vi "GETPINSTATUS.vi"(8 "error in (no error)":errorcluster, 9 "pin":dbl, 10 "Port":dbl, 11 "simulado in":refnum<class "simulado.lvclass">) -> (0 "error out":errorcluster, 3 "simulado out":refnum<class "simulado.lvclass">)   [LabVIEW 2019, in "simulado.lvclass"]
uses:
  simulado.lvclass
  simulado.lvclass/simulado.ctl
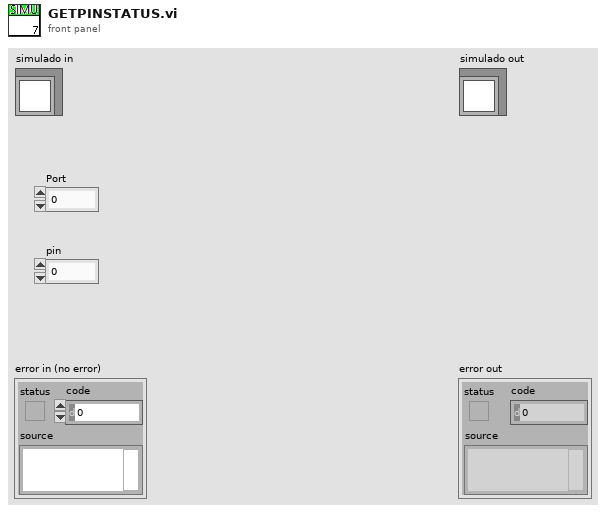
[diagram p1: front panel]
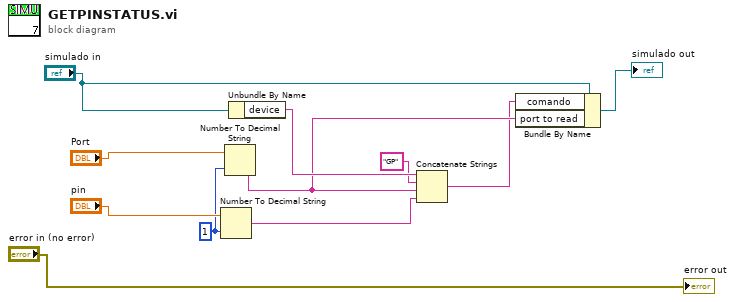
[diagram p0: block diagram]
diagram:
  w9 = i16 1 ("width (-)")
  n1 = Number To Decimal String(number="pin", width (-)=w9) -> (decimal integer string=w3:string)
  n2 = Number To Decimal String(number="Port", width (-)=w9) -> (decimal integer string=w4:string)
  n3 = Unbundle By Name("simulado in") -> ("device"=w6:string)
  n4 = Concatenate Strings(w6, "GP" ("string"), w4, w3) -> (w2:string)
  n5 = Bundle By Name(cluster="simulado in", "comando"=w2, "port to read"=w4) -> (→"simulado out":refnum<class "simulado.lvclass">)
  "error out" <- "error in (no error)"
